vi "GetSyncOption.vi"(5 "error in (no error)":errorcluster) -> (15 "SyncOption":T1, 17 "SyncTime(s)":i32, 19 "error out":errorcluster)   [LabVIEW 2014, in "UmlEditor.lvclass"]
uses:
  <resource>/Framework/Providers/Open_GDS/UML/UmlEditor_class/UmlEditor.lvclass
  <resource>/Framework/Providers/Open_GDS/UML/UMLEditor/UMLEditor_SyncOptions.ctl
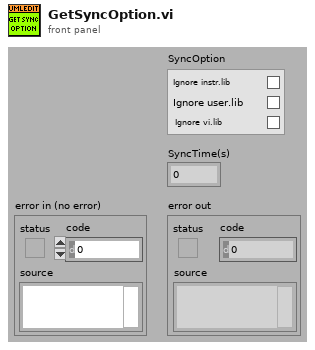
[diagram p1: front panel]
types:
  T1 = typedef "UMLEditor_SyncOptions.ctl" = cluster{"IgnoreInstrLib":bool, "IgnoreUserLib":bool, "IgnoreViLib":bool}
  T2 = typedef "UmlEditor.lvclass/ObjectAttributes.ctl" = cluster{"ListeningQueueIn":refnum<queue>, "Event":refnum<user-event>, "UseProjectFolderAsBasePath":bool, "TypeSyncOption":bool, "Attr":string[], "ToolTip":cluster{"ToolTipOpen":bool, "LastToolTip":i32}, "ClassesToIgnore":string[], "UndoSize":i32, "OpenLastSavedFileWhenStarting":bool, "SyncOption":T1, "SyncTime(s)":i32, "Params":cluster{"IniParams":T3, "Value":string}[], "GraphButtons":refnum<vi>}
  T3 = typedef "UmlEditor.lvclass/IniParamsType.ctl" = enum16{"I have problem with UML stability on my computer"}
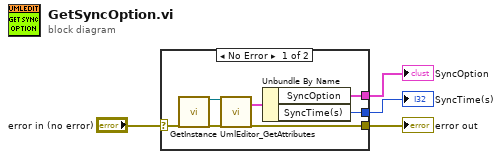
[diagram p0: block diagram]
diagram:
  n1 = case shown="No Error" "error in (no error)" {
    selector: "error in (no error)" -> [w7 w12]
    tunnel: [w11 w12] -> w3
    tunnel: [w10 _] -> w2
    tunnel: [w6 _] -> w1
    frame No Error {
      n2 = call <resource>:"GetInstance.vi"("error in (no error)"=w7) -> ("reference out"=w9:refnum<class "UmlEditor.lvclass">, "error out"=w8:errorcluster)  [unwired: 17 out]
      n3 = call <resource>:"UmlEditor_GetAttributes.vi"("reference in"=w9, "error in (no error)"=w8) -> ("Data"=w5:T2, "error out"=w11:errorcluster)  [unwired: 14 in, 2 out]
      n4 = Unbundle By Name(w5) -> ("SyncOption"=w10:T1, "SyncTime(s)"=w6:i32)
    }
    frame Error {
    }
  }
  "error out" <- w3
  "SyncOption" <- w2
  "SyncTime(s)" <- w1
